vi "scaler2.vi"(7 "L_k(t)":ext[][](array[numeric]), 11 "H_lk":ext[][][](array[numeric])) -> (3 "H_lk":ext[][][](array[numeric]))   [LabVIEW 2013]
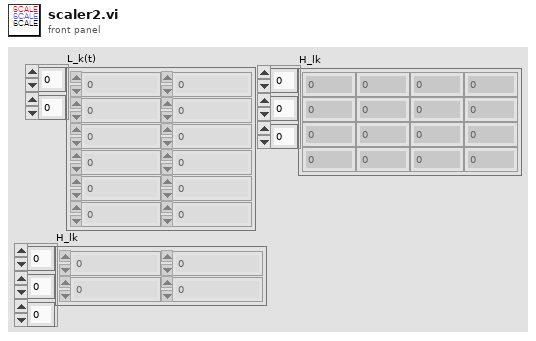
[diagram p1: front panel]
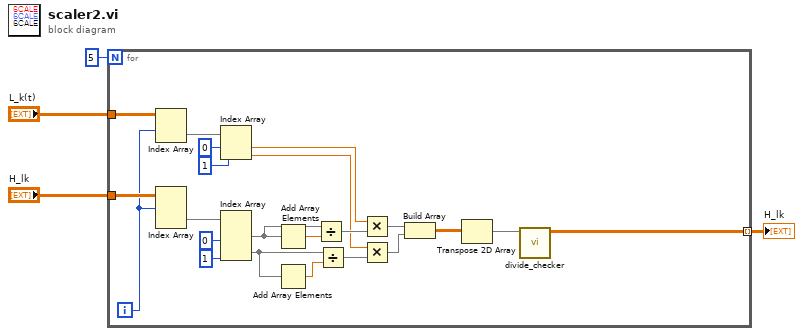
[diagram p0: block diagram]
diagram:
  n1 = for {
    N: 5 -> [_]
    tunnel: "L_k(t)" -> [w18]
    tunnel: "H_lk" -> [w26]
    tunnel: [w5] -> w1 mode=indexing
    i -> [w17]
    n2 = Index Array(array=w18, index (row)=w17) -> (element=w16:ext[])  [unwired: 1 in]
    n3 = Index Array(array=w26, index (dim 0)=w17) -> (element=w25:ext[][])  [unwired: 2 in]
    n4 = Index Array(array=w16, index #1=0 ("index"), index #2=1 ("index")) -> (element #1=w12:ext, element #2=w10:ext)
    n5 = Index Array(array=w25, index (col) #1=0 ("disabled index (col)"), index (col) #2=1 ("index (col)")) -> (element #1=w21:ext[], element #2=w20:ext[])  [unwired: 2 in]
    n6 = Add Array Elements(numeric array=w21) -> (sum=w22:ext)
    n7 = Add Array Elements(numeric array=w20) -> (sum=w19:ext)
    n8 = Divide(x=w21, y=w22) -> (x/y=w13:ext[])
    n9 = Divide(x=w20, y=w19) -> (x/y=w11:ext[])
    n10 = Multiply(x=w12, y=w13) -> (x*y=w9:ext[])
    n11 = Multiply(x=w10, y=w11) -> (x*y=w8:ext[])
    n12 = Build Array(w9, w8) -> (w7:ext[][])
    n13 = Transpose 2D Array(2D array=w7) -> (transposed array=w6:ext[][])
    n14 = call "divide_checker.vi"("H_lk"=w6) -> ("H_lk"=w5:ext[][])  [unwired: 10 in]
  }
  "H_lk" <- w1
